vi "Exercise 6_12__Read_Delimited_1D_Spreadsheet_file.vi"() -> ()   [LabVIEW 2018]
uses:
  <vilib>/Utility/file.llb/Read Delimited Spreadsheet (DBL).vi
panel:
  out "all rows":dbl[][](array[numeric]) caption="모든 행"
  out "웨이브폼 차트":dbl[](graph)
  out "first row":dbl[](array[numeric]) caption="첫번째 행"
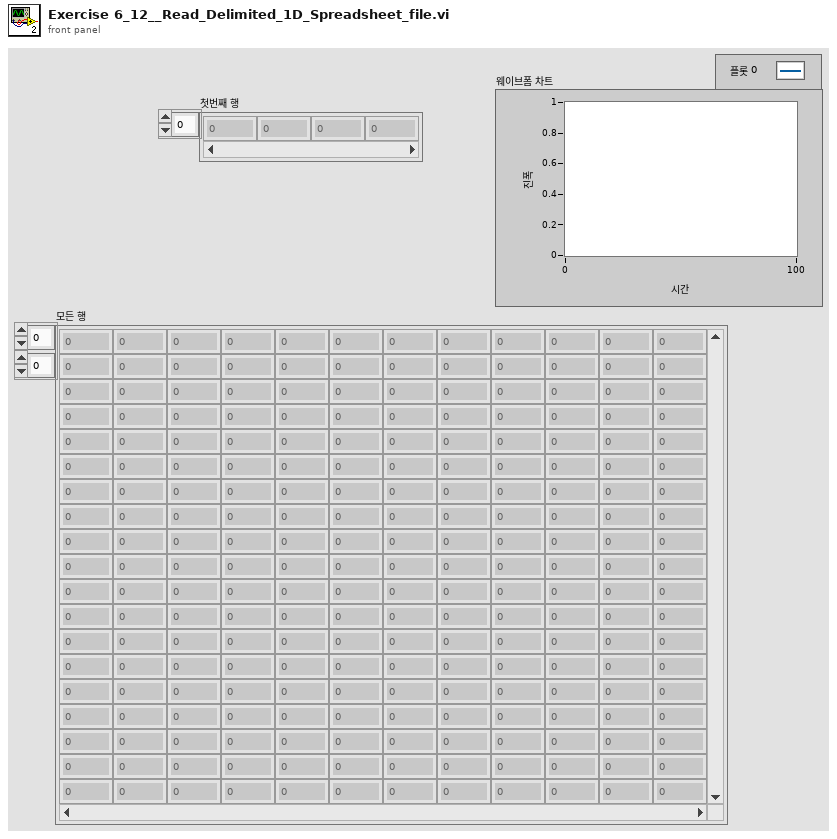
[diagram p1: front panel]
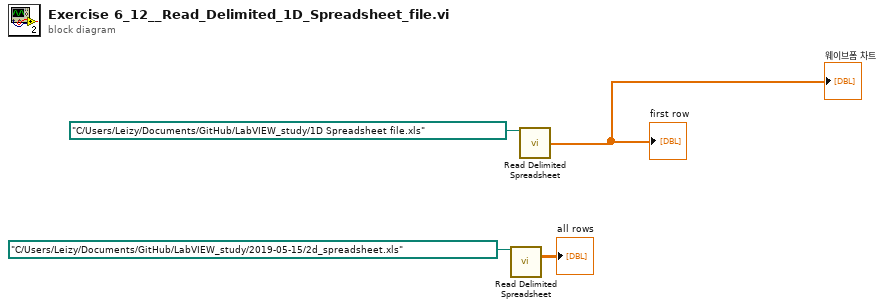
[diagram p0: block diagram]
diagram:
  n1 = call-poly <vilib>:"Read Delimited Spreadsheet.vi"("file path (dialog if empty)"=path "C:/Users/Leizy/Documents/GitHub/LabVIEW_study/2019-05-15/2d_spreadsheet.xls") -> ("all rows"=→"all rows":dbl[][])  [unwired: 9 in, 5 out]
  n2 = call-poly <vilib>:"Read Delimited Spreadsheet.vi"("file path (dialog if empty)"=path "C:/Users/Leizy/Documents/GitHub/LabVIEW_study/1D Spreadsheet file.xls") -> ("first row"=→"first row" →"웨이브폼 차트":dbl[])  [unwired: 9 in, 5 out]
